vi "security_decrypt.vi"(3 "FORMULA (if any)":string, 4 "METHOD":u16(ring) items=["#0_none", "#1_hexa", "#2_hexa_scrambled"], 6 "ENCRYPTED DATA":string) -> (0 "RAW DATA":string)   [LabVIEW 2018, in "db_lib R3.lvlib"]
uses:
  db_lib R3.lvlib
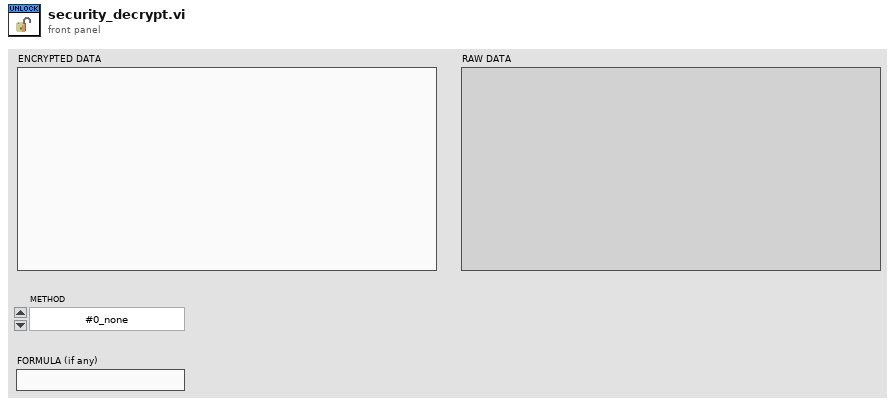
[diagram p1: front panel]
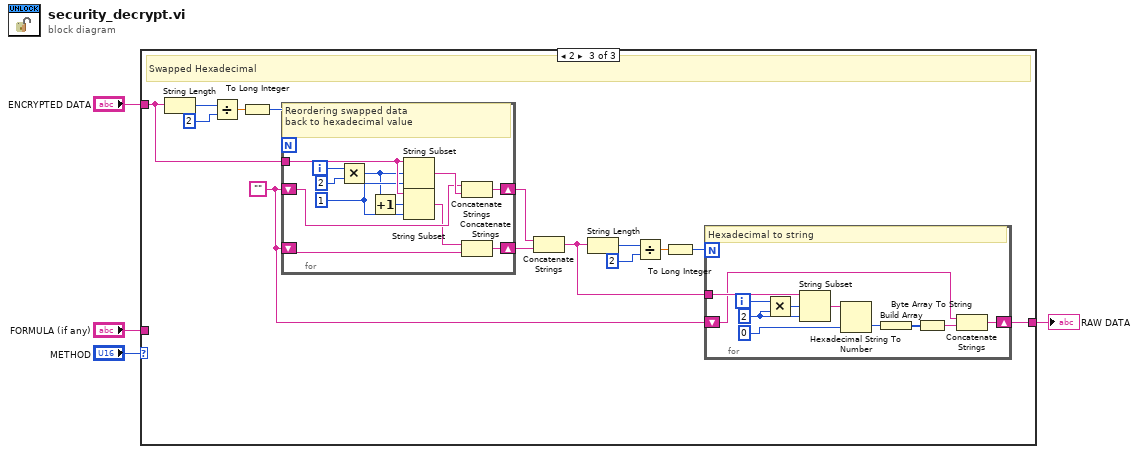
[diagram p0: block diagram]
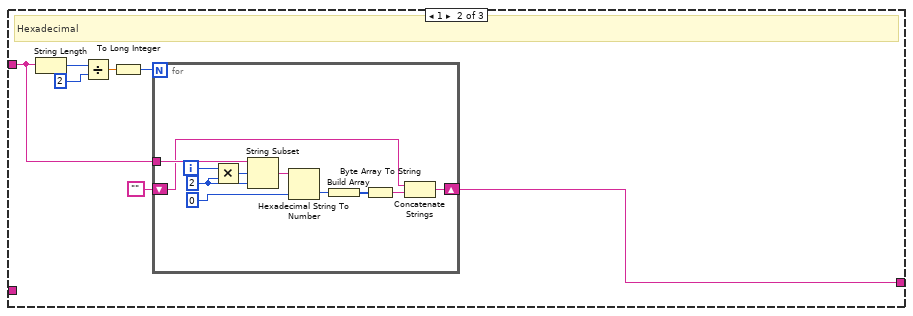
[diagram p3: hidden frame]
diagram:
  n1 = case shown="2" "METHOD" {
    tunnel: "FORMULA (if any)" -> [_ _ _]
    tunnel: "ENCRYPTED DATA" -> [w5 w8 w33]
    tunnel: [w5 w6 w24] -> w1
    frame 0, Default {
      # "None"
    }
    frame 1 {
      # "Hexadecimal"
      n2 = String Length(string=w8) -> (length=w12:i32)
      n3 = Divide(x=w12, y=2) -> (x/y=w10:dbl)
      n4 = To Long Integer(number=w10) -> (32bit integer=w9:i32)
      n5 = for {
        N: w9 -> [_]
        tunnel: w8 -> [w21]
        shift-right: [w15] -> w6
        shift-left: "" -> [w14]
        i -> [w23]
        w13 = 2 ("y")
        n6 = Multiply(x=w23, y=w13) -> (x*y=w22:i32)
        n7 = String Subset(string=w21, offset (0)=w22, length (rest)=w13) -> (substring=w20:string)
        n8 = Hexadecimal String To Number(string=w20, default (0uL)=u8 0 ("default (0 U32)")) -> (number=w18:u8)  [unwired: 1 in, 1 out]
        n9 = Build Array(w18) -> (w17:u8[])
        n10 = Byte Array To String(unsigned byte array=w17) -> (string=w16:string)
        n11 = Concatenate Strings(w14, w16) -> (w15:string)
      }
    }
    frame 2 {
      w25 = ""
      # "Swapped Hexadecimal"
      n12 = String Length(string=w33) -> (length=w37:i32)
      n13 = Divide(x=w37, y=2) -> (x/y=w35:dbl)
      n14 = To Long Integer(number=w35) -> (32bit integer=w34:i32)
      n15 = for {
        N: w34 -> [_]
        tunnel: w33 -> [w56]
        shift-right: [w60] -> w32
        shift-left: w25 -> [w52]
        shift-right: [w54] -> w31
        shift-left: w25 -> [w50]
        i -> [w58]
        w55 = u8 1 ("default (0 U32)")
        # "Reordering swapped data\nback to hexadecimal value"
        n16 = Multiply(x=w58, y=2) -> (x*y=w49:i32)
        n17 = Increment(x=w49) -> (x+1=w57:i32)
        n18 = String Subset(string=w56, offset (0)=w49, length (rest)=w55) -> (substring=w53:string)
        n19 = String Subset(string=w56, offset (0)=w57, length (rest)=w55) -> (substring=w51:string)
        n20 = Concatenate Strings(w52, w53) -> (w60:string)
        n21 = Concatenate Strings(w51, w50) -> (w54:string)
      }
      n22 = Concatenate Strings(w32, w31) -> (w26:string)
      n23 = String Length(string=w26) -> (length=w30:i32)
      n24 = Divide(x=w30, y=2) -> (x/y=w28:dbl)
      n25 = To Long Integer(number=w28) -> (32bit integer=w27:i32)
      n26 = for {
        N: w27 -> [_]
        tunnel: w26 -> [w46]
        shift-right: [w40] -> w24
        shift-left: w25 -> [w39]
        i -> [w48]
        w38 = 2 ("y")
        # "Hexadecimal to string"
        n27 = Multiply(x=w48, y=w38) -> (x*y=w47:i32)
        n28 = String Subset(string=w46, offset (0)=w47, length (rest)=w38) -> (substring=w45:string)
        n29 = Hexadecimal String To Number(string=w45, default (0uL)=u8 0 ("default (0 U32)")) -> (number=w43:u8)  [unwired: 1 in, 1 out]
        n30 = Build Array(w43) -> (w42:u8[])
        n31 = Byte Array To String(unsigned byte array=w42) -> (string=w41:string)
        n32 = Concatenate Strings(w39, w41) -> (w40:string)
      }
    }
  }
  "RAW DATA" <- w1
